vi "ModifyClassAttribute2.vi"(5 "error in (no error)":errorcluster) -> (19 "error out":errorcluster)   [LabVIEW 2010, in "G#SubSubClass1.lvclass"]
uses:
  G#SubSubClass1.lvclass
  G#SubClass1_class/G#SubClass1.lvclass
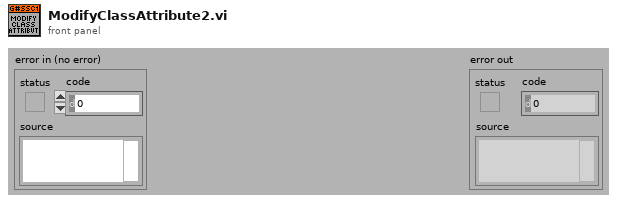
[diagram p1: front panel]
types:
  T1 = typedef "G#SubClass1.lvclass/ClassAttributesRef.ctl" = refnum<data-value>
  T2 = typedef "G#SubSubClass1.lvclass/ClassAttributesRef.ctl" = refnum<data-value>
  T3 = typedef "G#SubSubClass1.lvclass/ClassAttributes.ctl" = cluster{"SubSubIntAttribute":i32}
  T4 = typedef "G#SubClass1.lvclass/ClassAttributes.ctl" = cluster{"SubClassIntAttribute":i32}
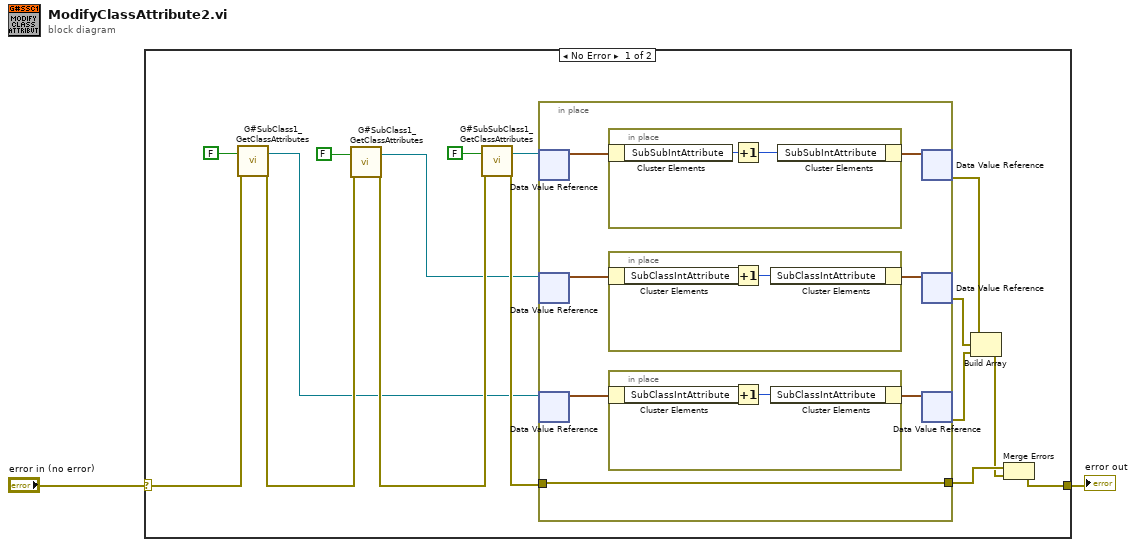
[diagram p0: block diagram]
diagram:
  n1 = case shown="No Error" "error in (no error)" {
    selector: "error in (no error)" -> [w11 w32]
    tunnel: [w16 w32] -> w1
    frame No Error {
      n2 = call "G#SubClass1_GetClassAttributes.vi"("return data? (T)"=FALSE ("return data"), "error in (no error)"=w11) -> ("class attributes ref"=w7:T1, "error out"=w10:errorcluster)  [unwired: 14 in, 2 out]
      n3 = call "G#SubClass1_GetClassAttributes.vi"("return data? (T)"=FALSE ("return data"), "error in (no error)"=w10) -> ("class attributes ref"=w8:T1, "error out"=w9:errorcluster)  [unwired: 14 in, 2 out]
      n4 = call "G#SubSubClass1_GetClassAttributes.vi"("return data? (T)"=FALSE ("return data"), "error in (no error)"=w9) -> ("class attributes ref"=w17:T2, "error out"=w18:errorcluster)  [unwired: 14 in, 2 out]
      n5 = in-place {
        in-place-border: w18 -> [w23]
        in-place-border: [w23] -> w14
        n6 = in-place-dvr #1(w17) -> (w24:T3)  [unwired: 1 out]
        n7 = in-place-dvr #2(w8) -> (w22:T4)  [unwired: 1 out]
        n8 = in-place-dvr #3(w7) -> (w21:T4)  [unwired: 1 out]
        n9 = in-place {
          n10 = in-place-cluster #4(w24) -> ("SubSubIntAttribute"=w31:i32)
          n11 = Increment(x=w31) -> (x+1=w30:i32)
          n12 = in-place-cluster #4("SubSubIntAttribute"=w30) -> (w25:T3)
        }
        n13 = in-place {
          n14 = in-place-cluster #5(w22) -> ("SubClassIntAttribute"=w29:i32)
          n15 = Increment(x=w29) -> (x+1=w28:i32)
          n16 = in-place-cluster #5("SubClassIntAttribute"=w28) -> (w20:T4)
        }
        n17 = in-place {
          n18 = in-place-cluster #6(w21) -> ("SubClassIntAttribute"=w27:i32)
          n19 = Increment(x=w27) -> (x+1=w26:i32)
          n20 = in-place-cluster #6("SubClassIntAttribute"=w26) -> (w19:T4)
        }
        n21 = in-place-dvr #1(w25) -> (w6:errorcluster)  [unwired: 1 out]
        n22 = in-place-dvr #2(w20) -> (w5:errorcluster)  [unwired: 1 out]
        n23 = in-place-dvr #3(w19) -> (w4:errorcluster)  [unwired: 1 out]
      }
      n24 = Build Array(w6, w5, w4) -> (w3:errorcluster[])
      n25 = Merge Errors(w14, w3) -> (w16:errorcluster)
    }
    frame Error {
    }
  }
  "error out" <- w1
